vi "get_lua_type.vi"(8 "error in (no error)":errorcluster, 11 "Lua in":refnum<class "Lua.lvclass">) -> (0 "error out":errorcluster, 2 "lua type":T1 items=["LUA_TNONE"=-1, "LUA_TNIL"=0, "LUA_TBOOLEAN"=1, "LUA_TLIGHTUSERDATA"=2, "LUA_TNUMBER"=3, "LUA_TSTRING"=4, "LUA_TTABLE"=5, "LUA_TFUNCTION"=6, "LUA_TUSERDATA"=7, "LUA_TTHREAD"=8, "LUA_NUMTYPES"=9], 3 "Lua out":refnum<class "Lua.lvclass">)   [LabVIEW 2020, in "Lua for LabVIEW.lvlib" / "Lua.lvclass"]
doc: "Returns the type of the value on top of the stack, or LUA_TNONE for a non-valid (but acceptable) index."
uses:
  Lua.lvclass
  Lua.lvclass/Lua.ctl
  lib/lua.dll/lua.dll.lvlib
  lib/lua.dll/lua_types.ctl
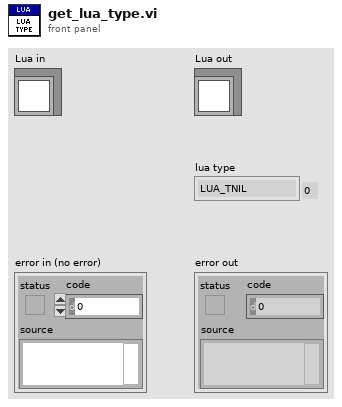
[diagram p1: front panel]
types:
  T1 = typedef "lua.dll.lvlib/lua_types.ctl" = i32
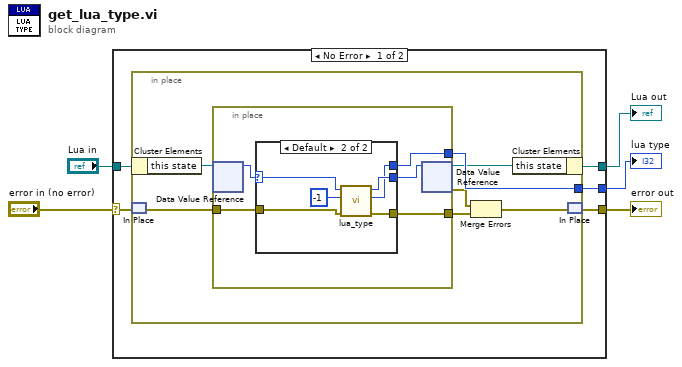
[diagram p0: block diagram]
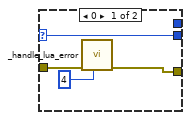
[diagram p2: hidden frame]
diagram:
  n1 = case shown="No Error" "error in (no error)" {
    selector: "error in (no error)" -> [w7 w34]
    tunnel: [w8 w34] -> w4
    tunnel: [w9 w33] -> w2
    tunnel: "Lua in" -> [w10 w33]
    tunnel: [w6 _] -> w1
    frame No Error {
      n2 = in-place {
        in-place-border: [w17] -> w6
        n3 = in-place-cluster #1(w10) -> ("this state"=w16:refnum<data-value>)
        n4 = in-place-match #2(w7) -> (w11:errorcluster)
        n5 = in-place {
          in-place-border: [w22] -> w17
          in-place-border: [w21] -> w13
          in-place-border: w11 -> [w20]
          n6 = in-place-dvr #3(w16) -> (w19:u64)  [unwired: 1 out]
          n7 = case shown="Default" w19 {
            selector: w19 -> [w26 w32]
            tunnel: [w26 w31] -> w18
            tunnel: w20 -> [w23 w29]
            tunnel: [w24 w28] -> w21
            tunnel: [_ w27] -> w22
            frame 0 {
              n8 = call "_handle_lua_error.vi"("lua status"=4 ("lua_load errcode"), "error in (no error)"=w23) -> ("error out"=w24:errorcluster)  [unwired: 9 in]
            }
            frame Default {
              n9 = call "lua_type.vi"("error in (no error)"=w29, "index"=-1, "lua_state_p"=w32) -> ("error out"=w28:errorcluster, "lua type"=w27:T1, "lua_state_p out"=w31:u64)  [unwired: 6 in]
            }
          }
          n10 = in-place-dvr #3(w18) -> (w15:refnum<data-value>, w14:errorcluster)
        }
        n11 = Merge Errors(w14, w13) -> (w12:errorcluster)
        n12 = in-place-cluster #1("this state"=w15) -> (w9:refnum<class "Lua.lvclass">)
        n13 = in-place-match #2(w12) -> (w8:errorcluster)
      }
    }
    frame Error {
    }
  }
  "error out" <- w4
  "Lua out" <- w2
  "lua type" <- w1
